vi "AE Ball Angle Distance.vi"(9 "Results 2":T1(array[cluster]) {"Normalized Center"."x" format="%#_2g"; "Normalized Center"."y" format="%#_2g"; "Overall Score" format="%#_2g"; "Distance (ft)" format="%#_3g"; "Area Score" format="%#_2g"; "Moment Score" format="%#_2g"; "Aspect Score" format="%#_2g"}, 11 "Port Angle":dbl) -> (3 "Port Angle Out":dbl)   [LabVIEW 2019]
uses:
  <vilib>/Rock Robotics/Network Tables/NT Write Number.vi
panel:
  out "Port Distance Out":dbl
  # "Scores"
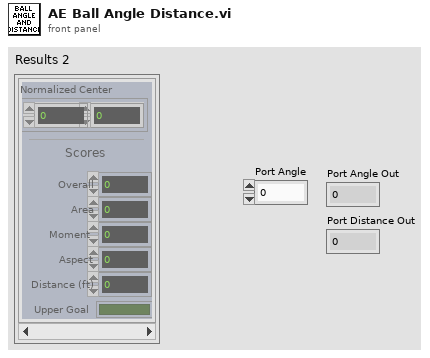
[diagram p1: front panel]
types:
  T1 = cluster{"diameter points":cluster{"first point":cluster{"x":dbl, "y":dbl}, "projected point":cluster{"x":dbl, "y":dbl}}, "Normalized Center":cluster{"x":dbl, "y":dbl}, "Overall Score":dbl, "Area Score":dbl, "Moment Score":dbl, "Aspect Score":dbl, "Distance (ft)":dbl, "Upper Goal":bool}[]
  T2 = cluster{"diameter points":cluster{"first point":cluster{"x":dbl, "y":dbl}, "projected point":cluster{"x":dbl, "y":dbl}}, "Normalized Center":cluster{"x":dbl, "y":dbl}, "Overall Score":dbl, "Area Score":dbl, "Moment Score":dbl, "Aspect Score":dbl, "Distance (ft)":dbl, "Upper Goal":bool}
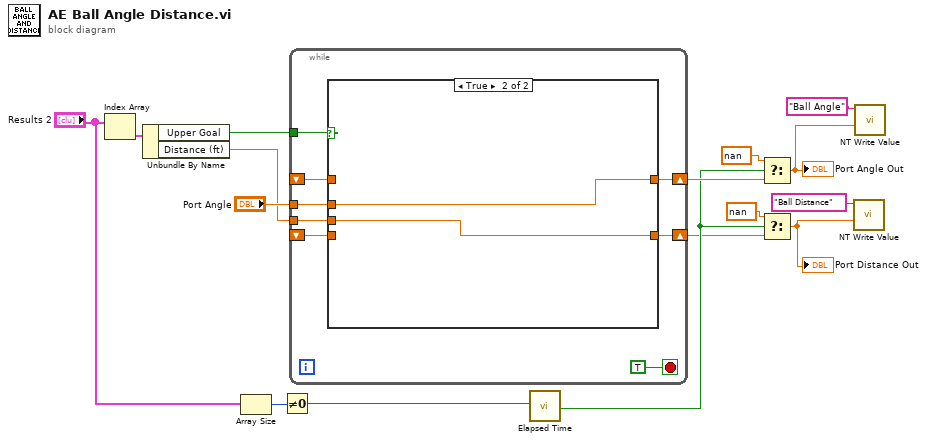
[diagram p0: block diagram]
diagram:
  n1 = Index Array(array="Results 2") -> (element=w15:T2)  [unwired: 1 in]
  n2 = Unbundle By Name(w15) -> ("Upper Goal"=w14:bool, "Distance (ft)"=w5:dbl)
  n3 = Array Size(array="Results 2") -> (size(s)=w12:i32)
  n4 = Not Equal To 0?(x=w12) -> (x != 0?=w10:bool)
  n5 = while {
    tunnel: w14 -> [w24]
    shift-right: [w23] -> w9
    shift-left: _ -> [w21]
    tunnel: "Port Angle" -> [w22]
    shift-right: [w18] -> w2
    shift-left: _ -> [w17]
    tunnel: w5 -> [w19]
    stop <- TRUE stop-if-true
    n6 = case shown="True" w24 {
      tunnel: [w26 w28] -> w23
      tunnel: w22 -> [_ w28]
      tunnel: w21 -> [w26 _]
      tunnel: w19 -> [_ w27]
      tunnel: [w25 w27] -> w18
      tunnel: w17 -> [w25 _]
      frame False {
      }
      frame True {
      }
    }
  }
  n7 = call "Elapsed Time"("Reset"=w10) -> ("Time has Elapsed"=w3:bool)  [unwired: 11 in, 7 out]
  n8 = Select(t=nan, s=w3, f=w9) -> (s? t:f=w7:dbl)
  "Port Angle Out" <- w7
  n9 = Select(t=nan, s=w3, f=w2) -> (s? t:f=w1:dbl)
  "Port Distance Out" <- w1
  n10 = call-poly <vilib>:"NT Write Value.vi"("Numeric"=w1, "Name"="Ball Distance") -> ()  [unwired: 9 in, 1 out]
  n11 = call-poly <vilib>:"NT Write Value.vi"("Numeric"=w7, "Name"="Ball Angle") -> ()  [unwired: 9 in, 1 out]
